vi "Monitor.vi"(0 "host name":string="higgsino.physics.ucsb.edu", 1 "binding key":string[](array[string])=["#"], 2 "queue name":string="monitor", 3 "error (in)":errorcluster, 4 "exchange name":u16(ring)=1 items=["requests", "alerts"]) -> (5 "Log":string, 6 "error out":errorcluster)   [LabVIEW 2016]
uses:
  C:/Program Files (x86)/National Instruments/LabVIEW 2016/vi.lib/Distrio/LabbitMQ/RabbitMQ.Client.dll
  Program Files (x86)/National Instruments/LabVIEW 2016/vi.lib/Distrio/LabbitMQ/RabbitMQ.Client.dll
  <vilib>/Distrio/LabbitMQ/Queue/Queue.lvclass
  <vilib>/Distrio/LabbitMQ/Connection/Connection.lvclass
panel:
  in  "stop":bool
  in  "Tab Control":enum32{"AMQP Settings", "Logger"}(tab)
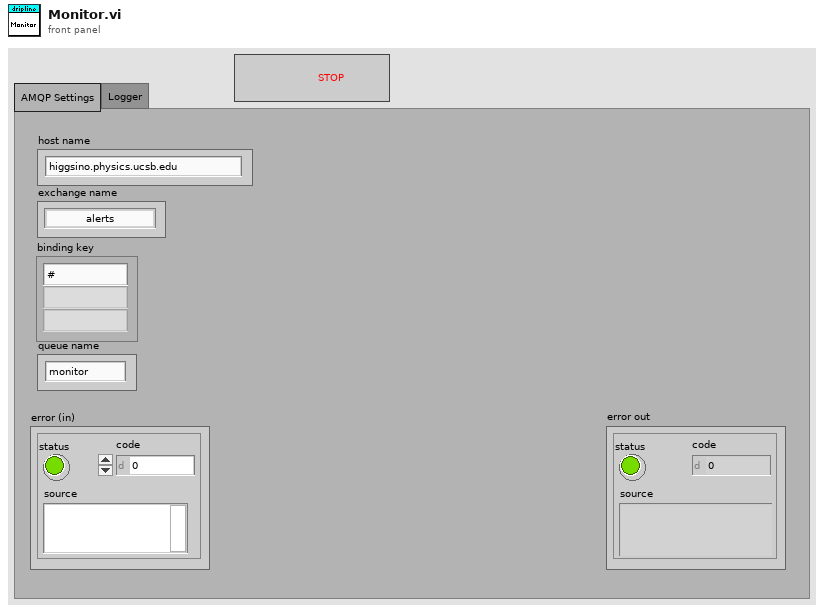
[diagram p1: front panel]
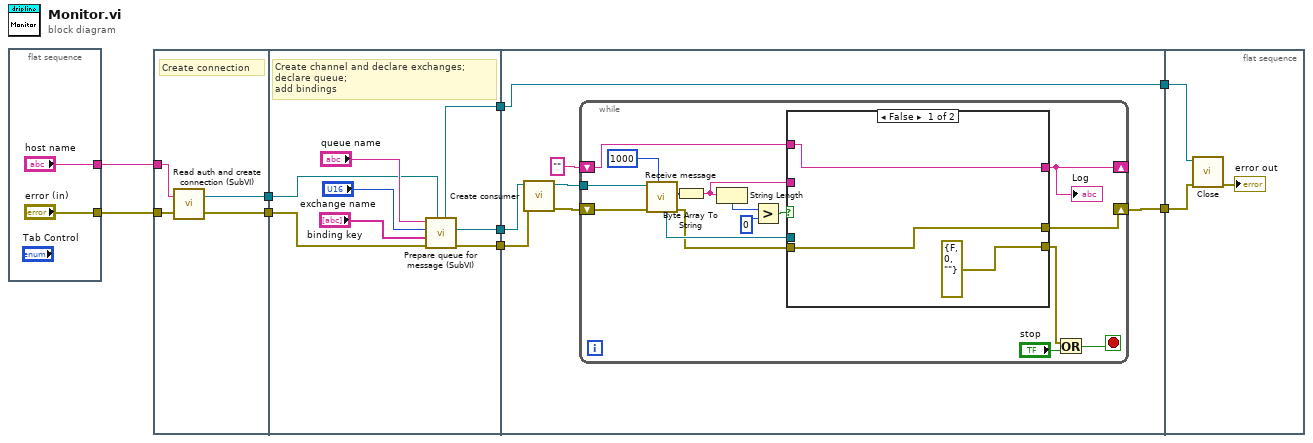
[diagram p0: block diagram]
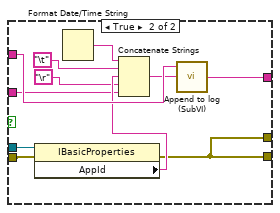
[diagram p2: hidden frame]
diagram:
  n1 = flat-sequence {
    tunnel: ["error (in)"] -> w7
    tunnel: ["host name"] -> w6
    frame #0 {
    }
  }
  n2 = flat-sequence {
    tunnel: [w13] -> w9
    tunnel: [w12] -> w8
    tunnel: w6 -> [w15]
    tunnel: w7 -> [w14]
    tunnel: w9 -> [w18]
    tunnel: w8 -> [w17]
    tunnel: [w20] -> w4
    tunnel: [w19] -> w3
    tunnel: [w16] -> w1
    tunnel: [w29] -> w5
    tunnel: w4 -> [w26]
    tunnel: w3 -> [w25]
    tunnel: [w24] -> w2
    tunnel: w1 -> [w24]
    tunnel: w5 -> [w62]
    tunnel: w2 -> [w61]
    frame #0 {
      # "Create connection"
      n3 = call "Read auth and create connection (SubVI).vi"("error in (no error)"=w14, "host name"=w15) -> ("error out"=w12:errorcluster, "Connection out"=w13:refnum<class "Connection.lvclass">)
    }
    frame #1 {
      # "Create channel and declare exchanges; declare queue;\nadd bindings"
      n4 = call "Prepare queue for message (SubVI).vi"("Connection in"=w18, "error in (no error)"=w17, "binding key"="binding key", "exchange name"="exchange name", "queue \nname"="queue name") -> ("error out"=w19:errorcluster, "Queue out"=w20:refnum<class "Queue.lvclass">, "Connection out"=w16:refnum<class "Connection.lvclass">)  [unwired: 2 out]
    }
    frame #2 {
      n5 = call <vilib>:"Create consumer.vi"("error in (no error)"=w25, "Queue in"=w26) -> ("error out"=w28:errorcluster, "Queue out"=w30:refnum<class "Queue.lvclass">)  [unwired: 8 in]
      n6 = while {
        tunnel: w30 -> [w46]
        shift-right: [w38] -> w29
        shift-left: w28 -> [w45]
        shift-right: [w42] -> _
        shift-left: "" -> [w43]
        stop <- w31 stop-if-true
        n7 = call <vilib>:"Receive message.vi"("millisecondsTimeout"=1000, "error in (no error)"=w45, "Consumer in"=w46) -> ("error out"=w40:errorcluster, "message body"=w44:u8[], "MessageProperties"=w41:refnum<k24>)  [unwired: 3 in, 3 out]
        n8 = Byte Array To String(unsigned byte array=w44) -> (string=w32:string)
        n9 = String Length(string=w32) -> (length=w35:i32)
        n10 = Greater?(x=w35, y=0) -> (0:w33:bool)
        n11 = case shown="False" w33 {
          tunnel: w43 -> [w49 w60]
          tunnel: [w49 w59] -> w42
          tunnel: w41 -> [_ w58]
          tunnel: w32 -> [_ w53]
          tunnel: w40 -> [w48 w51]
          tunnel: [w48 w50] -> w38
          tunnel: [errorcluster {"status"=FALSE, "code"=0, "source"=""} ("error out") w50] -> w37
          frame False {
          }
          frame True {
            n12 = property class="IBasicProperties"(reference=w58, error in=w51) -> (error out=w50:errorcluster, "AppId"=w55:string)  [unwired: 1 out]
            n13 = Format Date/Time String() -> (date/time string=w57:string)  [unwired: 3 in]
            n14 = Concatenate Strings(w57, "\t", w55, "\r", w53) -> (w52:string)
            n15 = call "Append to log (SubVI).vi"("to append"=w52, "log in"=w60) -> ("log out"=w59:string)  [unwired: 1 in]
          }
        }
        "Log" <- w42
        n16 = Or(x=w37, y="stop") -> (x .or. y?=w31:bool)
      }
    }
    frame #3 {
      n17 = call <vilib>:"Close.vi"("error in (no error)"=w62, "Connection in"=w61) -> ("error out"=→"error out":errorcluster)  [unwired: 8 in, 1 out]
    }
  }
